vi "Point Test Shapes.vi"(7 "Array":cluster{"Time (s)":dbl, T1, bool}[](array[cluster]), 9 "Coords":T3, 10 "Points":cluster{"x":dbl, "y":dbl, "th":dbl}[](array[cluster]), 11 "Picture in":refnum<vi>) -> (2 "Pt Test Results":enum16{"Miss", "Rect Hit", "Arrow Hit"}(ring), 3 "Results":T4)   [LabVIEW 2019]
uses:
  <vilib>/Utility/miscctls.llb/LVPoint32TypeDef.ctl
  Command Stuff/Single Cmd Info.ctl
  <vilib>/picture/picture.llb/imagedata.ctl
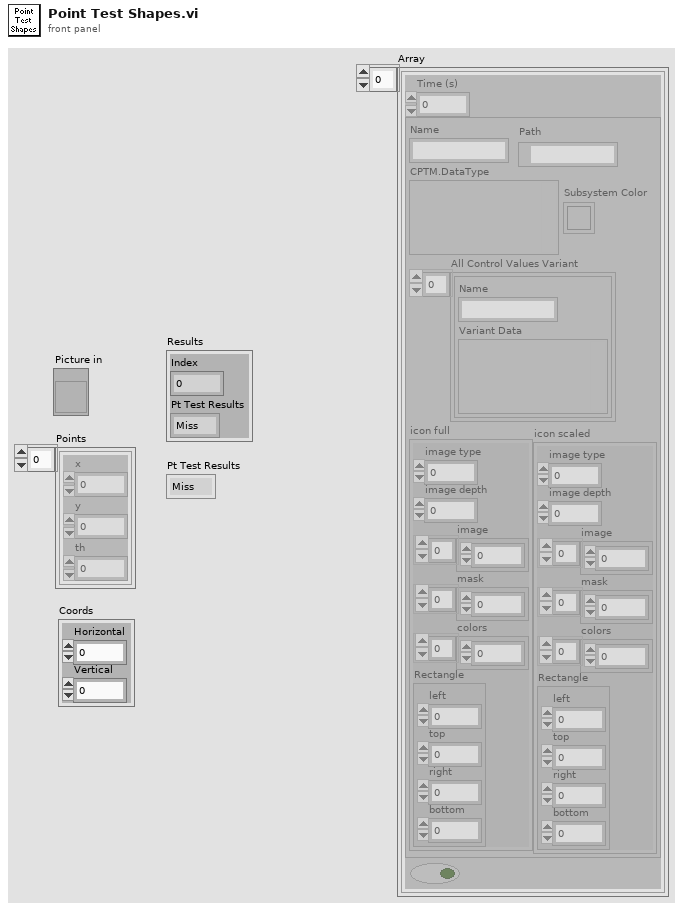
[diagram p1: front panel]
types:
  T1 = typedef "Single Cmd Info.ctl" = cluster{"Name":string, "CPTM.DataType":variant, "All Control Values Variant":cluster{"Name":string, "Variant Data":variant}[], "icon full":T2, "icon scaled":T2, "Path":path, "Subsystem Color":u32}
  T2 = typedef "imagedata.ctl" = cluster{"image type":i32, "image depth":i32, "image":u8[], "mask":u8[], "colors":u32[], "Rectangle":cluster{"left":i16, "top":i16, "right":i16, "bottom":i16}}
  T3 = typedef "LVPoint32TypeDef.ctl" = cluster{"Horizontal":i32, "Vertical":i32}
  T4 = cluster{"Index":i32, "Pt Test Results":enum16{"Miss", "Rect Hit", "Arrow Hit"}}
  T5 = cluster{i32, "Pt Test Results":enum16{"Miss", "Rect Hit", "Arrow Hit"}}
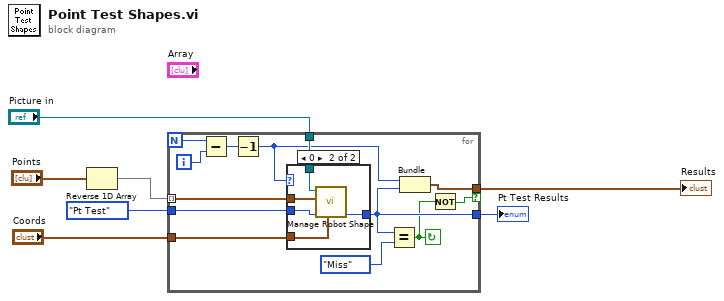
[diagram p0: block diagram]
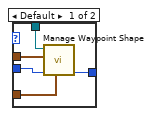
[diagram p2: hidden frame]
diagram:
  n1 = Reverse 1D Array(array="Points") -> (reversed array=w1:cluster{"x":dbl, "y":dbl, "th":dbl}[])
  n2 = for {
    N -> [w11]
    tunnel: "Coords" -> [w20]
    tunnel: "Picture in" -> [w19]
    tunnel: [w16] -> w5
    tunnel: enum16{"Draw", "Pt Test"}."Pt Test" ("Operation") -> [w18]
    tunnel: w1 -> [w17] mode=indexing
    tunnel: [w14] -> w7 if=w13
    i -> [w10]
    stop <- w12 continue-if-true
    n3 = Subtract(x=w11, y=w10) -> (x-y=w9:i32)
    n4 = Decrement(x=w9) -> (x-1=w8:i32)
    n5 = case shown="0" w8 {
      tunnel: w20 -> [w22 w30]
      tunnel: w19 -> [w25 w29]
      tunnel: [w21 w28] -> w16
      tunnel: w18 -> [w23 w27]
      tunnel: w17 -> [w24 w26]
      frame Default {
        n6 = call "Manage Waypoint Shape.vi"("Coords"=w22, "Operation"=w23, "Waypoint Position (ft)"=w24, "Pict Ref"=w25) -> ("Pt Test Results"=w21:enum16{"Miss", "Rect Hit", "Arrow Hit"})  [unwired: 6 in, 1 out]
      }
      frame 0 {
        n7 = call "Manage Robot Shape.vi"("Coords"=w30, "Operation"=w27, "Robot Position (ft)"=w26, "Pict Ref"=w29) -> ("Pt Test Results"=w28:enum16{"Miss", "Rect Hit", "Arrow Hit"})  [unwired: 5 in, 2 out]
      }
    }
    n8 = Equal?(x=w16, y=enum16{"Miss", "Rect Hit", "Arrow Hit"}."Miss" ("Pt Test Results")) -> (x = y?=w12:bool)
    n9 = Bundle(w8, "Pt Test Results"=w16) -> (w14:T5)  [unwired: 1 in]
    n10 = Not(x=w12) -> (.not. x?=w13:bool)
  }
  "Results" <- w7
  "Pt Test Results" <- w5
